vi "Get Siblings.vi"(0 "Tree Reference In":refnum<vi>, 2 "Input Tag (Current)":string, 5 "error in (no error)":errorcluster) -> (14 "Tree Reference Out":refnum<vi>, 16 "Sibling Tags":string[](array[string]), 19 "error out":errorcluster)   [LabVIEW 2011, in "VITesterUtilities.lvlib"]
doc: "Retrieves a 1-D array of tags of all items in the tree that have the same parent and deletes the requested tag giving all siblings of an item. Uses the currently selected item if the tag input is unwired."
uses:
  Libraries/VITesterUtilities.lvlib
panel:
  # "VI INPUTS"
  # "VI OUTPUTS"
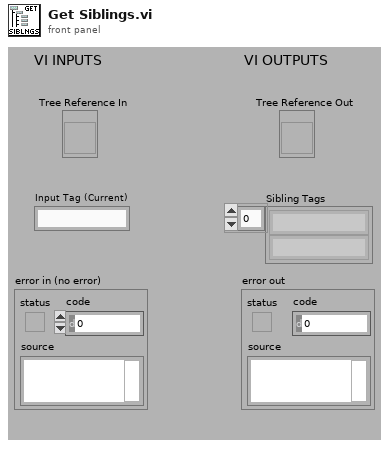
[diagram p1: front panel]
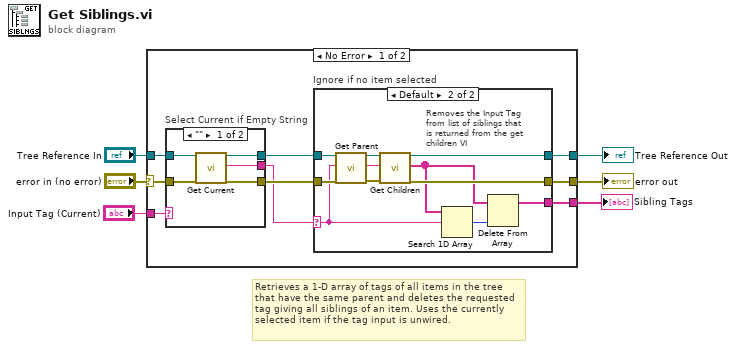
[diagram p0: block diagram]
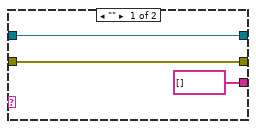
[diagram p2: hidden frame]
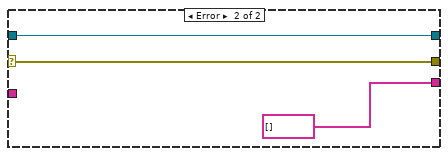
[diagram p4: hidden frame]
diagram:
  # "Retrieves a 1-D array of tags of all items in the tree that have the same parent and deletes the requested tag giving all siblings of an item. Uses the currently selected item if the tag input is unwired."
  n1 = case shown="No Error" "error in (no error)" {
    selector: "error in (no error)" -> [w10 w39]
    tunnel: "Tree Reference In" -> [w12 w40]
    tunnel: "Input Tag (Current)" -> [w8 _]
    tunnel: [w15 w40] -> w4
    tunnel: [w13 string[] []] -> w3
    tunnel: [w14 w39] -> w2
    frame No Error {
      n2 = case "Select Current if Empty String" shown="\"\"" w8 {
        selector: w8 -> [_ w35]
        tunnel: [w33 w37] -> w11
        tunnel: w12 -> [w34 w37]
        tunnel: [w32 w36] -> w9
        tunnel: w10 -> [w31 w36]
        tunnel: [w30 w35] -> w7
        frame "" {
          n3 = call "Get Current.vi"("Tree Reference In"=w34, "error in (no error)"=w31) -> ("Tree Reference Out"=w33:refnum<vi>, "Current Tag"=w30:string, "error out"=w32:errorcluster)  [unwired: 14 in, 1 out]
        }
        frame Default {
        }
      }
      n4 = case "Ignore if no item selected" shown="Default" w7 {
        selector: w7 -> [_ w19]
        tunnel: [w18 w26] -> w15
        tunnel: [w17 w25] -> w14
        tunnel: [string[] [] ("Children Tags") w23] -> w13
        tunnel: w11 -> [w18 w22]
        tunnel: w9 -> [w17 w21]
        frame "" {
        }
        frame Default {
          # "Removes the Input Tag from list of siblings that is returned from the get children VI"
          n5 = call "Get Parent.vi"("Tree Reference In"=w22, "Child Tag (Current)"=w19, "error in (no error)"=w21) -> ("Tree Reference Out"=w29:refnum<vi>, "Parent Tag"=w28:string, "error out"=w27:errorcluster)  [unwired: 13 in, 1 out]
          n6 = call "Get Children.vi"("Tree Reference In"=w29, "Parent Tag"=w28, "error in (no error)"=w27) -> ("Tree Reference Out"=w26:refnum<vi>, "Children Tags"=w20:string[], "error out"=w25:errorcluster)  [unwired: 14 in]
          n7 = Search 1D Array(1D array=w20, element=w19) -> (index of element=w24:i32)  [unwired: 1 in]
          n8 = Delete From Array(array=w20, index=w24) -> (array with subset deleted=w23:string[])  [unwired: 1 in, 1 out]
        }
      }
    }
    frame Error {
    }
  }
  "Sibling Tags" <- w3
  "Tree Reference Out" <- w4
  "error out" <- w2
